vi "header.vi"() -> (3 "concatenated string":string)   [LabVIEW 2017]
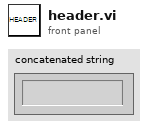
[diagram p1: front panel]
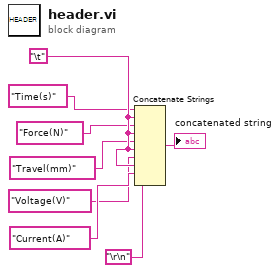
[diagram p0: block diagram]
diagram:
  w7 = "\t"
  n1 = Concatenate Strings("Time(s)", w7, "Force(N)", w7, "Travel(mm)", w7, "Voltage(V)", w7, "Current(A)", "\r\n") -> (→"concatenated string":string)
